vi "Ready_measurement.vi"(9 "String":string="*RST;:SYST:ZCH ON;:FUNC \"CHAR\";CHAR:RANG:AUTO ON;:SYST:ZCH OFF;:CALC2:NULL:STAT ON", 11 "VISA resource name":refnum<visa-resource-name>="COM4") -> ()   [LabVIEW 2024]
uses:
  support/Serial - XON-XOFF Characters.ctl
  support/Serial - ASCII Characters.ctl
  support/Serial - Settings.ctl
  <vilib>/Instr/_visa.llb/VISA Configure Serial Port (Instr).vi
panel:
  # "• When the path pointer detects a colon (:), it moves down to the next command level. An exception is when the path pointer detects a semicolon (;), which is used to separate commands within the program message. \n• When the path pointer detects a colon (:) that immediately follows a semicolon (;), it resets to the root level. \n• The path pointer can only move down. It cannot be moved up a level. Executing a command at a higher level requires that you start over at the root command."
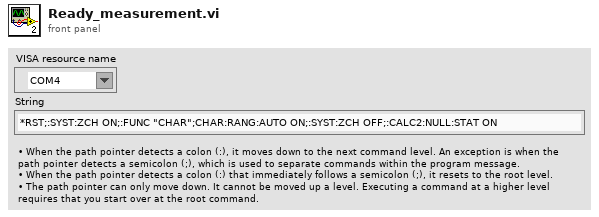
[diagram p1: front panel]
types:
  T1 = typedef "Serial - Settings.ctl" = cluster{"baud rate":u32, "data bits":u16, "parity":enum16{"None", "Odd", "Even", "Mark", "Space"}, "stop bits":u16, "flow control":u16}
  T2 = typedef "Serial - XON-XOFF Characters.ctl" = cluster{"XON":T3, "XOFF":T3}
  T3 = typedef "Serial - ASCII Characters.ctl" = enum16{"NUL", "SOH", "STX", "ETX", "EOT", "ENQ", "ACK", "BEL", "BS", "HT", "LF", "VT", "FF", "CR", "SO", "SI", "DLE", "DC1", "DC2", "DC3", "DC4", "NAK", "SYN", "ETB", "CAN", "EM", "SUB", "ESC", "FS", "GS", "RS", "US", "SP", "!", "\"", "#", "$", "%", "&", "'", "(", ")", "*", "+", ",", "- (-)", ".", "/", "0", "1", "2", "3", "4", "5", "6", "7", "8", "9", ":", ";", "<", "=", ">", "?", "@", "A", "B", "C", "D", "E", "F", "G", "H", "I", "J", "K", "L", "M", "N", "O", "P", "Q", "R", "S", "T", "U", "V", "W", "X", "Y", "Z", "[", "\\", "]", "^", "_", "`", "a", "b", "c", "d", "e", "f", "g", "h", "i", "j", "k", "l", "m", "n", "o", "p", "q", "r", "s", "t", "u", "v", "w", "x", "y", "z", "{", "|", "}", "~"}
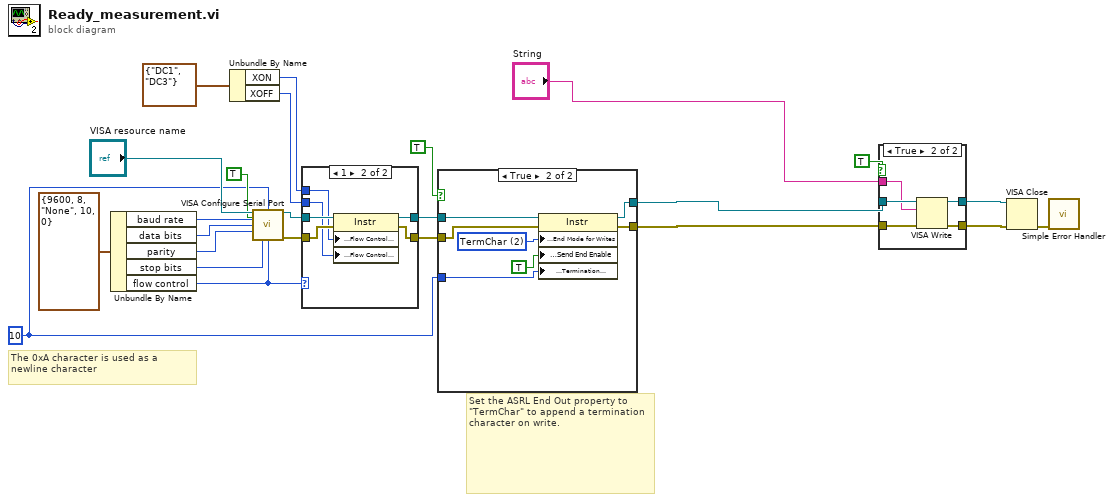
[diagram p0: block diagram]
diagram:
  w8 = u8 10 ("Termination Character")
  # "The 0xA character is used as a newline character"
  # "Set the ASRL End Out property to \"TermChar\" to append a termination character on write."
  n1 = Unbundle By Name(T1 {"baud rate"=9600, "data bits"=8, "parity"=enum."None", "stop bits"=10, "flow control"=0} ("Serial Settings")) -> ("baud rate"=w17:u32, "data bits"=w18:u16, "parity"=w19:enum16{"None", "Odd", "Even", "Mark", "Space"}, "stop bits"=w20:u16, "flow control"=w14:u16)
  n2 = Unbundle By Name(T2 {"XON"=enum."DC1", "XOFF"=enum."DC3"} ("XON/XOFF Characters")) -> ("XON"=w13:T3, "XOFF"=w12:T3)
  n3 = call-poly "VISA Configure Serial Port"("VISA resource name"="VISA resource name", "termination char\n(0xA = '\\n' = LF)"=w8, "Enable Termination\nChar (T)"=TRUE ("End Read on Termination Character?"), "baud rate (9600)"=w17, "data bits (8)"=w18, "parity (0:none)"=w19, "stop bits (10: 1 bit)"=w20, "flow control (0:none)"=w14) -> ("VISA resource name out"=w21:refnum<visa-resource-name>, "error out"=w22:errorcluster)  [unwired: 2 in, 4 out]
  n4 = case shown="1" w14 {
    tunnel: [w25 w32] -> w11
    tunnel: [w26 w31] -> w10
    tunnel: w22 -> [w25 w30]
    tunnel: w21 -> [w26 w29]
    tunnel: w13 -> [_ w28]
    tunnel: w12 -> [_ w27]
    frame Default {
    }
    frame 1 {
      n5 = property class="Instr"(reference=w29, error in=w30, "Serial Settings:Flow Control XON Character"=w28, "Serial Settings:Flow Control XOFF Character"=w27) -> (reference out=w31:refnum<visa-resource-name>, error out=w32:errorcluster)
    }
  }
  n6 = case shown="True" TRUE ("End Write on Termination Character?") {
    tunnel: w10 -> [w33 w41]
    tunnel: w11 -> [w34 w40]
    tunnel: [w33 w39] -> w4
    tunnel: [w34 w38] -> w3
    tunnel: w8 -> [_ w36]
    frame False {
    }
    frame True {
      w37 = u16 2 items=["None", "LastBit", "TermChar", "Break"] ("Serial Settings:Serial End Mode for Writes")
      n7 = property class="Instr"(reference=w41, error in=w40, "Serial Settings:End Mode for Writes"=w37, "Message Based Settings:Send End Enable"=TRUE, "Message Based Settings:Termination Character"=w36) -> (reference out=w39:refnum<visa-resource-name>, error out=w38:errorcluster)
    }
  }
  n8 = case shown="True" TRUE {
    tunnel: w4 -> [w43 w48]
    tunnel: w3 -> [w42 w47]
    tunnel: [w43 w46] -> w5
    tunnel: [w42 w45] -> w6
    tunnel: "String" -> [_ w44]
    frame False {
    }
    frame True {
      n9 = VISA Write(VISA resource name=w48, write buffer=w44, error in (no error)=w47) -> (VISA resource name out=w46:refnum<visa-resource-name>, error out=w45:errorcluster)  [unwired: 1 out]
    }
  }
  n10 = VISA Close(VISA resource name=w5, error in (no error)=w6) -> (error out=w7:errorcluster)
  n11 = call <vilib>:"Simple Error Handler.vi"("error in (no error)"=w7) -> ()  [unwired: 1 in, 8 out]
